vi "WPI_GyroGetAngle.vi"(8 "error in (no error)":errorcluster, 11 "GyroDevRef":T1={"DevStatus"={"status"=FALSE, "code"=0, "source"=""}, "Analog Channel"=enum."AI 1", "Gain (VoltsPerDegree/Second)"=0.0, "Gyro Type"=enum."Analog", "Handle"=0, "SPI Bus"=enum."Invalid", "Device Found"=FALSE, "Sample Rate"=1.0, "Calibrate On Open"=FALSE, "Offset"=0.0} {"Sample Rate" min=0.25 max=100.0 step=0.25}) -> (0 "error out":errorcluster, 1 "Angular Rate":dbl, 2 "Angle":dbl, 3 "GyroDevRef":T1={"DevStatus"={"status"=FALSE, "code"=0, "source"=""}, "Analog Channel"=enum."AI 1", "Gain (VoltsPerDegree/Second)"=0.0, "Gyro Type"=enum."Analog", "Handle"=0, "SPI Bus"=enum."Invalid", "Device Found"=FALSE, "Sample Rate"=1.0, "Calibrate On Open"=FALSE, "Offset"=0.0} {"Sample Rate" min=0.25 max=100.0 step=0.25})   [LabVIEW 2017]
doc: "Returns the angle, in degrees, from the original heading that the robot is currently facing.\n\nThis software is licensed. Open the labview\\readme\\WPI Robotics Library Open Source License.txt file for more information."
uses:
  <vilib>/Rock Robotics/WPI/Gyro/WPI_GyroDevRef.ctl
  <vilib>/Rock Robotics/SystemInterfaces/AI/FPGA_AIChannel.ctl
  <vilib>/Rock Robotics/SystemInterfaces/spilib/spi_bus.ctl
  <vilib>/Rock Robotics/SystemInterfaces/AI/FPGA_AIGyroChannel.ctl
  <instrlib>/Sparkfun Atomic IMU/HAIOL/Sparkfun Atomic IMU.lvclass
  <instrlib>/Honeywell Compass HMC6343/HAIOL/Honeywell Compass HMC6343.lvclass
panel:
  # "Analog"
  # "XRS"
  # "Analog"
  # "XRS"
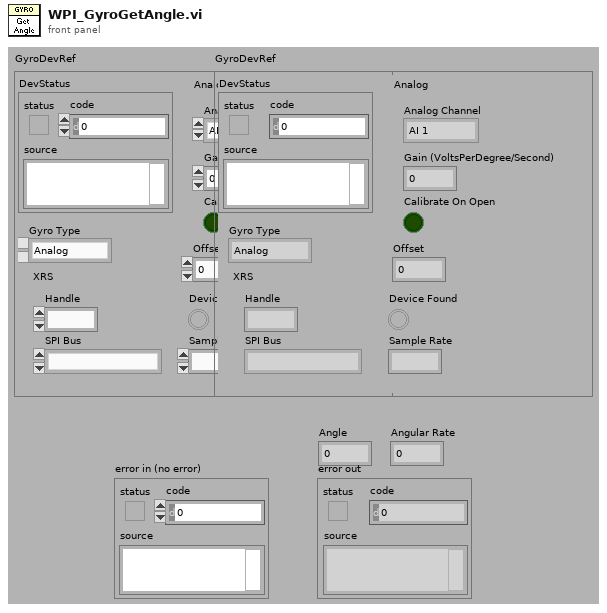
[diagram p1: front panel]
types:
  T1 = typedef "WPI_GyroDevRef.ctl" = cluster{"DevStatus":errorcluster, "Analog Channel":T2, "Gain (VoltsPerDegree/Second)":dbl, "Gyro Type":enum16{"Analog", "XRS450"}, "Handle":i32, "SPI Bus":T3, "Device Found":bool, "Sample Rate":dbl, "Calibrate On Open":bool, "Offset":dbl}
  T2 = typedef "FPGA_AIChannel.ctl" = enum8{"AI 0", "AI 1", "AI 2", "AI 3", "AI MXP 0", "AI MXP 1", "AI MXP 2", "AI MXP 3", "Invalid"}
  T3 = typedef "spi_bus.ctl" = enum16{"SPI On-Board, CS0", "SPI On-Board, CS1", "SPI On-Board, CS2", "SPI On-Board, CS3", "SPI MXP", "Invalid"}
  T4 = typedef "FPGA_AIGyroChannel.ctl" = enum8{"AI 0", "AI 1", "Invalid"}
  T5 = cluster{"Pitch (deg/s)":dbl, "Roll (deg/s)":dbl, "Yaw (deg/s)":dbl}
  T6 = cluster{"Head (deg)":dbl, "Pitch (deg)":dbl, "Roll (deg)":dbl}
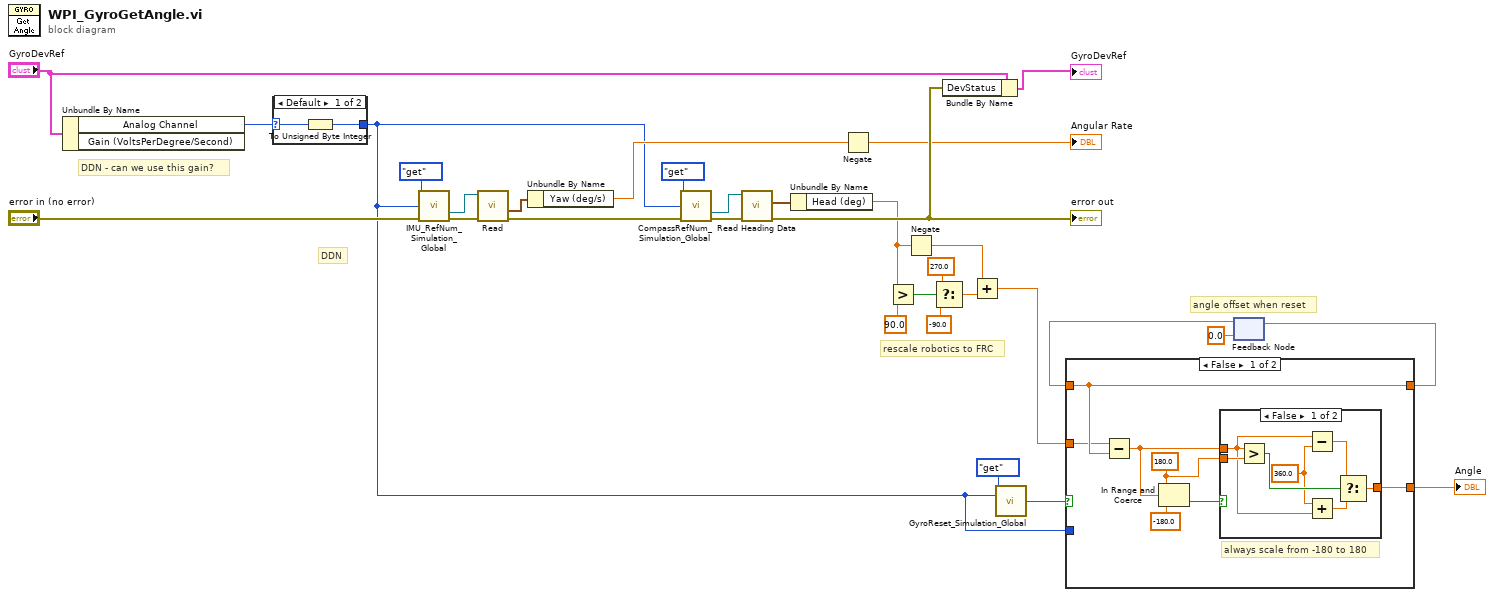
[diagram p0: block diagram]
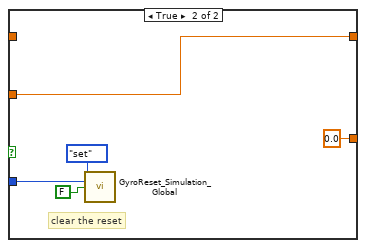
[diagram p3: hidden frame]
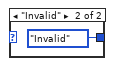
[diagram p4: hidden frame]
diagram:
  # "angle offset when reset"
  # "rescale robotics to FRC"
  # "DDN"
  # "DDN - can we use this gain?"
  n1 = Unbundle By Name("GyroDevRef") -> ("Analog Channel"=w28:T2)  [unwired: 1 out]
  n2 = case shown="Default" w28 {
    selector: w28 -> [w33 _]
    tunnel: [w32 FPGA_AIGyroChannel."Invalid" ("Analog Channel")] -> w1
    frame Default {
      n3 = To Unsigned Byte Integer(number=w33) -> (unsigned 8bit integer=w32:u8)
    }
    frame "Invalid" {
    }
  }
  n4 = call <vilib>:"IMU_RefNum_Simulation_Global.vi"("menu"=enum16{"set", "get", "delete"}."get", "Analog Channel"=w1, "error in (no error)"="error in (no error)") -> ("Sparkfun Atomic IMU Get"=w25:refnum<class "Sparkfun Atomic IMU.lvclass">, "error out"=w26:errorcluster)  [unwired: 11 in]
  n5 = call-dynamic "Read.vi"("error in (no error)"=w26, "Sparkfun Atomic IMU in"=w25) -> ("error out"=w22:errorcluster, "Gyros Data"=w24:T5)  [unwired: 6 in, 2 out]
  n6 = Unbundle By Name(w24) -> ("Yaw (deg/s)"=w23:dbl)
  n7 = call <vilib>:"CompassRefNum_Simulation_Global.vi"("menu"=enum16{"set", "get", "delete"}."get", "Analog Channel"=w1, "error in (no error)"=w22) -> ("Honeywell Compass HMC6343 Get"=w17:refnum<class "Honeywell Compass HMC6343.lvclass">, "error out"=w19:errorcluster)  [unwired: 11 in]
  n8 = call-dynamic "Read Heading Data.vi"("error in (no error)"=w19, "Honeywell Compass HMC6343"=w17) -> ("error out"=w21:errorcluster, "Heading Data"=w18:T6)  [unwired: 7 in, 1 out]
  "error out" <- w21
  n9 = Unbundle By Name(w18) -> ("Head (deg)"=w9:dbl)
  n10 = Negate(x=w23) -> (-x=→"Angular Rate":dbl)
  n11 = Greater?(x=w9, y=90.0) -> (0:w14:bool)
  n12 = Negate(x=w9) -> (-x=w12:dbl)
  n13 = Select(t=270.0, s=w14, f=-90.0) -> (s? t:f=w13:dbl)
  n14 = Bundle By Name(cluster="GyroDevRef", "DevStatus"=w21) -> (→"GyroDevRef":T1)
  n15 = Add(x=w12, y=w13) -> (x+y=w3:dbl)
  n16 = call <vilib>:"GyroReset_Simulation_Global.vi"("menu"=enum16{"set", "get", "delete"}."get", "Gyro Channel"=w1) -> ("reset out"=w7:bool)  [unwired: 12 in, 1 out]
  n17 = feedback #1(0.0 ("In Gauge")) -> (w5:dbl)
  n18 = case shown="False" w7 {
    tunnel: w5 -> [w37 _]
    tunnel: [w37 w54] -> w4
    tunnel: w3 -> [w36 w54]
    tunnel: [w35 0.0] -> w2
    tunnel: w1 -> [_ w51]
    frame False {
      w41 = 180.0 ("y")
      # "always scale from -180 to 180"
      n19 = Subtract(x=w36, y=w37) -> (x-y=w38:dbl)
      n20 = In Range and Coerce(upper limit=w41, x=w38, lower limit=-180.0 ("y")) -> (In Range?=w40:bool)  [unwired: 1 out]
      n21 = case shown="False" w40 {
        tunnel: [w47 w49] -> w35
        tunnel: w38 -> [w43 w49]
        tunnel: w41 -> [w48 _]
        frame False {
          w42 = 360.0 ("y")
          n22 = Greater?(x=w43, y=w48) -> (0:w46:bool)
          n23 = Subtract(x=w43, y=w42) -> (x-y=w45:dbl)
          n24 = Add(x=w42, y=w43) -> (x+y=w44:dbl)
          n25 = Select(t=w45, s=w46, f=w44) -> (s? t:f=w47:dbl)
        }
        frame True {
        }
      }
    }
    frame True {
      # "clear the reset"
      n26 = call <vilib>:"GyroReset_Simulation_Global.vi"("menu"=enum16{"set", "get", "delete"}."set", "Gyro Channel"=w51, "reset in"=FALSE) -> ()  [unwired: 11 in, 2 out]
    }
  }
  "Angle" <- w2
  n27 = feedback-in #1(w4) -> ()
